vi "Test Subset.vi"() -> ()   [LabVIEW 2024, in "Spectrum Recorder too.lvclass"]
uses:
  Spectrum Recorder too.lvclass
  Spectrum Recorder too.lvclass/Spectrum Recorder too.ctl
panel:
  out "Output subset pointer 2":i32
  out "Output subset":dbl[](array[numeric])
  in  "Output subset length":i32
  in  "Output subset pointer":i32
  in  "Output values":dbl[](array[numeric])=[1.0, 2.0, 3.0, 4.0]
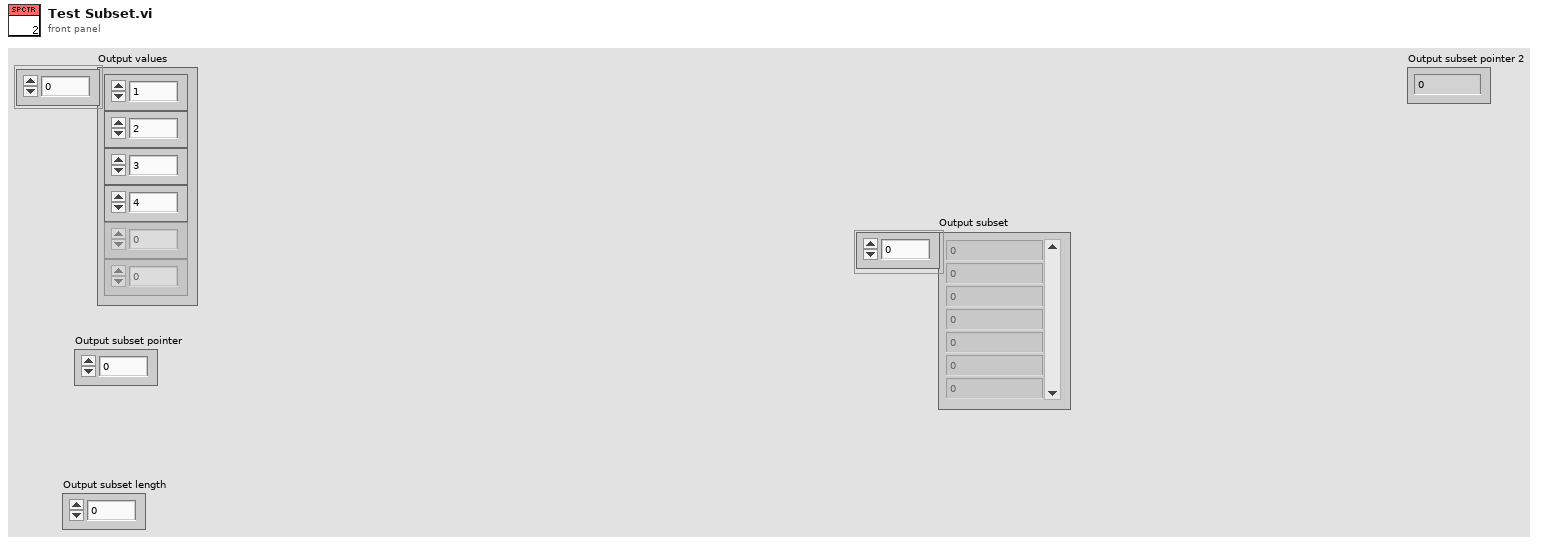
[diagram p1: front panel]
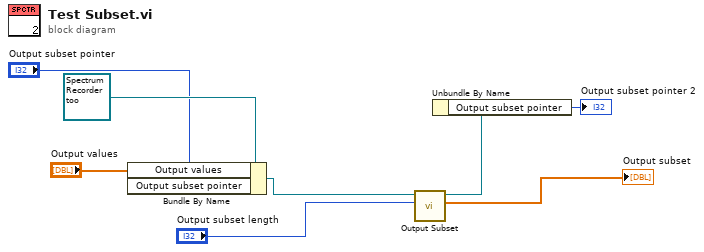
[diagram p0: block diagram]
diagram:
  n1 = Bundle By Name(cluster=refnum<class "Spectrum Recorder too.lvclass"> refnum ("Spectrum Recorder too.lvclass"), "Output values"="Output values", "Output subset pointer"="Output subset pointer") -> (w5:refnum<class "Spectrum Recorder too.lvclass">)
  n2 = call-dynamic "Output Subset.vi"("Output subset length"="Output subset length", "Spectrum Recorder too in"=w5) -> ("Output subset"=→"Output subset":dbl[], "Spectrum Recorder too out"=w2:refnum<class "Spectrum Recorder too.lvclass">)  [unwired: 7 in, 1 out]
  n3 = Unbundle By Name(w2) -> ("Output subset pointer"=→"Output subset pointer 2":i32)
